vi "Stream Output Values.vi"(7 "Motor List":T1[](array[typedef]), 10 "Drive Velocity Values":dbl[](array[numeric]), 11 "Drive Velocity Times":dbl[](array[numeric])) -> ()   [LabVIEW 2020, in "SwerveDrive_ACT.lvlib"]
uses:
  SwerveDrive_ACT.lvlib
  Shared Code/TypeDefs/ENUM_Motor Index.ctl
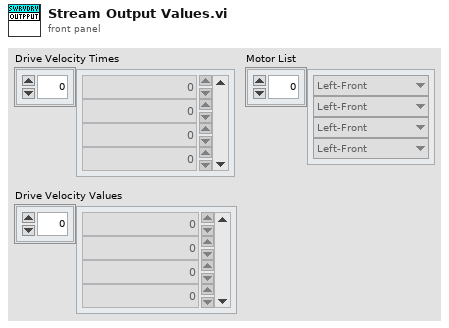
[diagram p1: front panel]
types:
  T1 = typedef "ENUM_Motor Index.ctl" = enum16{"Left-Front", "Right-Front", "Left-Back", "Right-Back"}
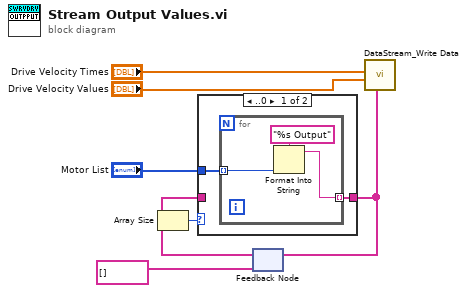
[diagram p0: block diagram]
diagram:
  n1 = feedback #1(string[] []) -> (w3:string[])
  n2 = Array Size(array=w3) -> (size(s)=w4:i32)
  n3 = case shown="..0" w4 {
    tunnel: w3 -> [_ w13]
    tunnel: [w8 w13] -> w2
    tunnel: "Motor List" -> [w9 _]
    frame ..0 {
      n4 = for {
        tunnel: w9 -> [w12] mode=indexing
        tunnel: [w10] -> w8 mode=indexing
        n5 = Format Into String(format string="%s Output", w12) -> (resulting string=w10:string)  [unwired: 2 in, 1 out]
      }
    }
    frame 1.. {
    }
  }
  n6 = feedback-in #1(w2) -> ()
  n7 = call "DataStream_Write Data.vi"("Header Array"=w2, "Value Array"="Drive Velocity Values", "Time Stamp Array"="Drive Velocity Times") -> ()  [unwired: 7 in, 2 out]
